vi "Close.vi"(8 "Error In":errorcluster, 11 "Display Manager In":refnum<class "Display Manager.lvclass">) -> (0 "Error Out":errorcluster)   [LabVIEW 2019, in "Display Manager.lvclass"]
uses:
  Display Manager.lvclass
  Process/Process.lvclass
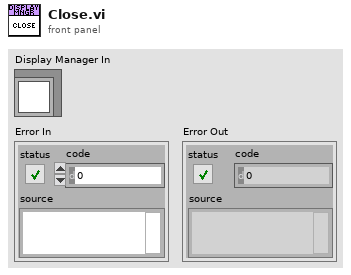
[diagram p1: front panel]
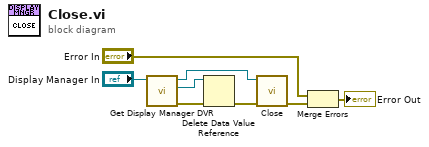
[diagram p0: block diagram]
diagram:
  n1 = call "Get Display Manager DVR.vi"("Display Manager In"="Display Manager In") -> ("Error Out"=w5:errorcluster, "DVR"=w6:refnum<data-value>, "Display Manager Out"=w4:refnum<class "Display Manager.lvclass">)  [unwired: 8 in]
  n2 = Delete Data Value Reference(data value reference=w6, error in=w5) -> (error out=w1:errorcluster)  [unwired: 1 out]
  n3 = call-parent "Close.vi"("Error In"=w1, "Process In"=w4) -> ("Error Out"=w8:errorcluster)  [unwired: 9 in]
  n4 = Merge Errors("Error In", w8) -> (→"Error Out":errorcluster)
